vi "Find Item By Tag.vi"(10 "Tag":string, 11 "Item List":T1) -> (3 "Item Info":T2)   [LabVIEW 2021]
uses:
  Control/Item Info.ctl
  Control/Item List.ctl
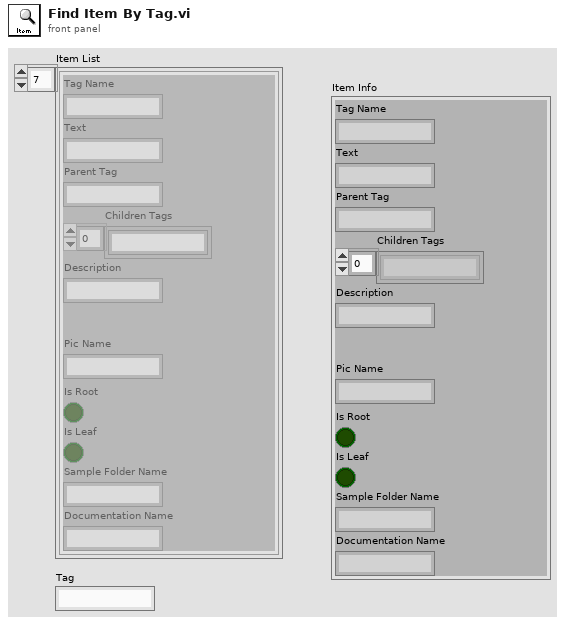
[diagram p1: front panel]
types:
  T1 = typedef "Item List.ctl" = T2[]
  T2 = typedef "Item Info.ctl" = cluster{"Tag Name":string, "Text":string, "Parent Tag":string, "Children Tags":string[], "Description":string, "Pic Name":string, "Is Root":bool, "Is Leaf":bool, "Sample Folder Name":string, "Documentation Name":string}
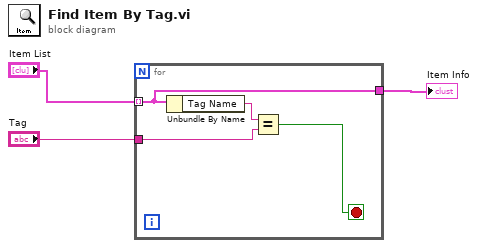
[diagram p0: block diagram]
diagram:
  n1 = for {
    tunnel: "Item List" -> [w4] mode=indexing
    tunnel: "Tag" -> [w6]
    tunnel: [w4] -> w3
    stop <- w5 stop-if-true
    n2 = Unbundle By Name(w4) -> ("Tag Name"=w7:string)
    n3 = Equal?(x=w7, y=w6) -> (x = y?=w5:bool)
  }
  "Item Info" <- w3
